vi "PID Target Angle.vi"() -> ()   [LabVIEW 2014]
panel:
  out "PID Target Angle":dbl
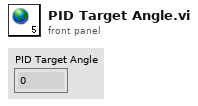
[diagram p1: front panel]
diagram:
